vi "Determine Warnings 4-1.vi"(8 "error in (no error)":errorcluster, 9 "Min Temp":dbl, 10 "Max Temp":dbl, 11 "Current Temp":dbl) -> (0 "error out":errorcluster, 1 "Warning?":bool, 2 "Warning Text":string)   [LabVIEW 2014]
doc: "This VI will determine whether a temperature warning is needed based on the current, minimum, and maximum temperatures being inputted. \nInputs: Current Temp, Max Temp, Min Temp\nOutputs: Warning Text, Warning?\nEmma Gordon\n9/8/16"
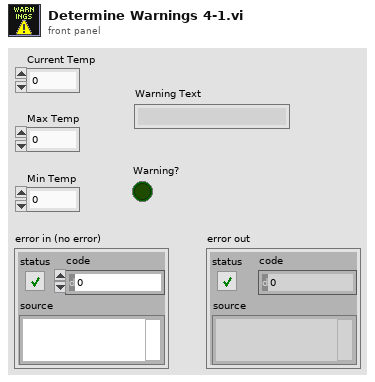
[diagram p1: front panel]
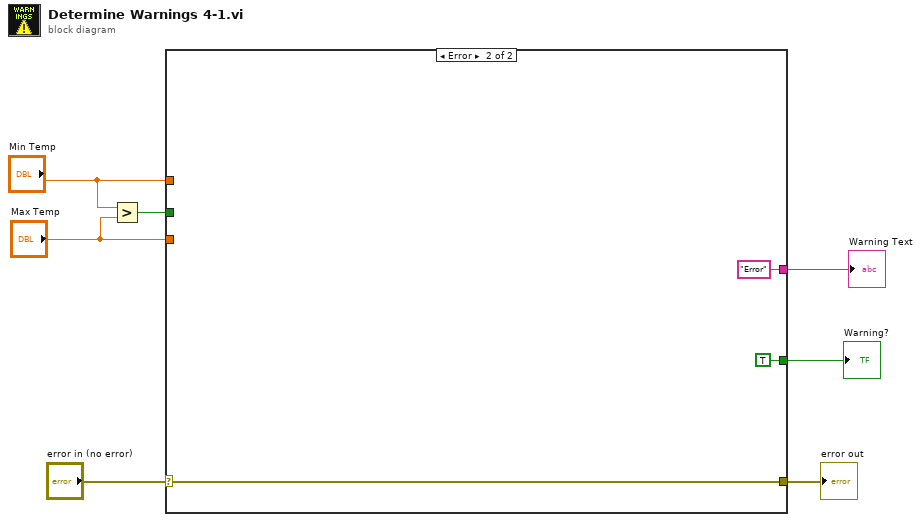
[diagram p0: block diagram]
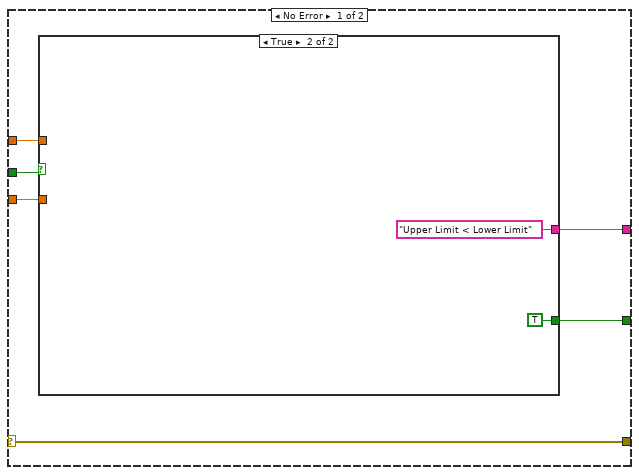
[diagram p2: hidden frame]
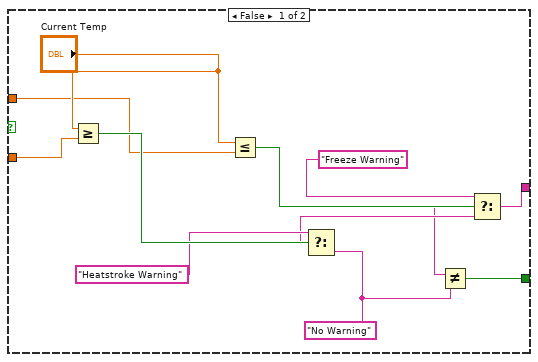
[diagram p3: hidden frame]
diagram:
  n1 = Greater?(x="Min Temp", y="Max Temp") -> (0:w3:bool)
  n2 = case shown="Error" "error in (no error)" {
    selector: "error in (no error)" -> [w8 w29]
    tunnel: [w13 "Error"] -> w7
    tunnel: [w12 TRUE] -> w6
    tunnel: "Min Temp" -> [w11 _]
    tunnel: "Max Temp" -> [w10 _]
    tunnel: w3 -> [w9 _]
    tunnel: [w8 w29] -> w1
    frame No Error {
      n3 = case shown="True" w9 {
        tunnel: [w18 "Upper Limit < Lower Limit"] -> w13
        tunnel: [w16 TRUE] -> w12
        tunnel: w11 -> [w15 _]
        tunnel: w10 -> [w14 _]
        frame False {
          w17 = "No Warning"
          n4 = Greater Or Equal?(x="Current Temp", y=w14) -> (x >= y?=w23:bool)
          n5 = Less Or Equal?(x="Current Temp", y=w15) -> (x <= y?=w21:bool)
          n6 = Select(t="Heatstroke Warning", s=w23, f=w17) -> (s? t:f=w19:string)
          n7 = Select(t="Freeze Warning", s=w21, f=w19) -> (s? t:f=w18:string)
          n8 = Not Equal?(x=w18, y=w17) -> (x != y?=w16:bool)
        }
        frame True {
        }
      }
    }
    frame Error {
    }
  }
  "Warning Text" <- w7
  "Warning?" <- w6
  "error out" <- w1
